vi "FRCts20_Backend_Test_Comment_GET.vi"(8 "error in (no error)":errorcluster, 11 "Note Index":u32) -> (0 "error out":errorcluster, 1 "Time (ms)":u32, 2 "Status":string, 3 "Note Out":T1, 5 "Success":bool)   [LabVIEW 2013, in "FRCts20_Backend_TestCode.lvlib"]
uses:
  FRCts20_Backend_TestCode.lvlib
  FRCts20_Backend_API/FRCts20_Backend_API_Note.ctl
  FRCts20_Backend_API/FRCts20_Backend_API_Command_Note.ctl
  FRCts20_Backend_API/FRCts20_Backend_API_Comment.vi
  FRCts20_Backend_API/FRCts20_Backend_API.lvlib
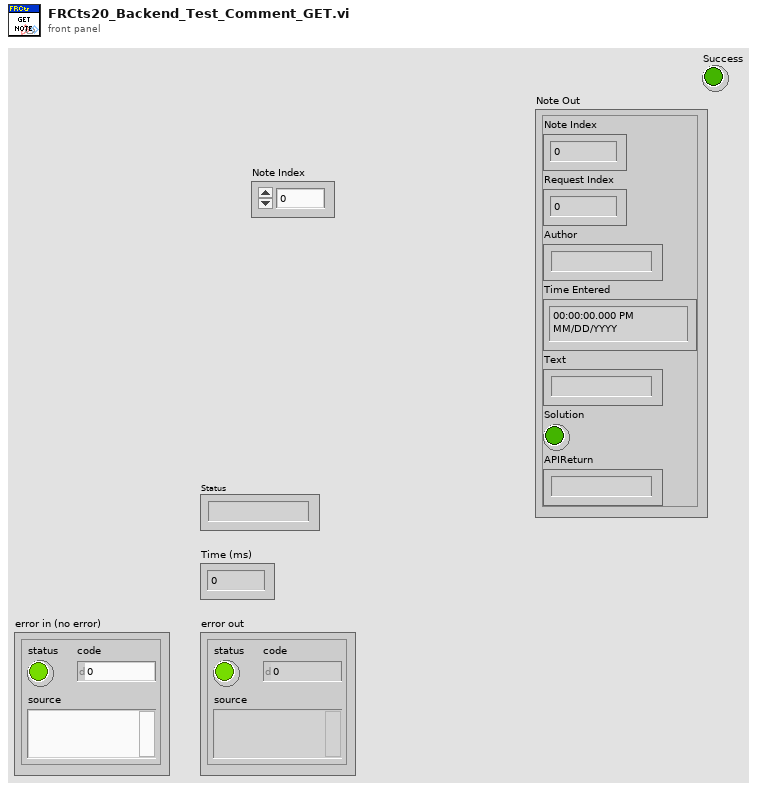
[diagram p1: front panel]
types:
  T1 = typedef "FRCts20_Backend_API.lvlib/FRCts20_Backend_API_Note.ctl" = cluster{"Note Index":u32, "Request Index":u32, "Author":string, "Time Entered":timestamp, "Text":string, "Solution":bool, "APIReturn":string}
  T2 = typedef "FRCts20_Backend_API.lvlib/FRCts20_Backend_API_Command_Note.ctl" = string
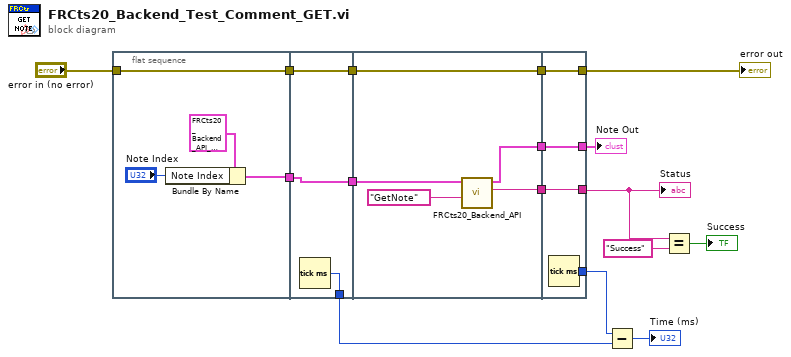
[diagram p0: block diagram]
diagram:
  n1 = flat-sequence {
    tunnel: [w20] -> w16
    tunnel: "error in (no error)" -> [w19]
    tunnel: [w19] -> w15
    tunnel: w16 -> [w21]
    tunnel: [w23] -> w8
    tunnel: [w22] -> w14
    tunnel: w15 -> [w22]
    tunnel: [w21] -> w2
    tunnel: [w28] -> w13
    tunnel: [w27] -> w12
    tunnel: [w26] -> w11
    tunnel: w14 -> [w26]
    tunnel: w2 -> [w24]
    tunnel: w13 -> [w32]
    tunnel: w12 -> [w31]
    tunnel: [w32] -> w5
    tunnel: [w31] -> w1
    tunnel: [w30] -> w7
    tunnel: [w29] -> w10
    tunnel: w11 -> [w29]
    frame #0 {
      n2 = Bundle By Name(cluster=T1 {"Note Index"=0, "Request Index"=0, "Author"="", "Time Entered"=timestamp(0 s since 1904-01-01), "Text"="", "Solution"=FALSE, "APIReturn"=""} ("Note In"), "Note Index"="Note Index") -> (w20:T1)
    }
    frame #1 {
      n3 = Tick Count (ms)() -> (millisecond timer value=w23:u32)
    }
    frame #2 {
      n4 = call-poly "FRCts20_Backend_API.vi"("Command"=T2 "GetNote", "Note In"=w24) -> ("Status"=w28:string, "Note Out"=w27:T1)  [unwired: 7 in, 1 out]
    }
    frame #3 {
      n5 = Tick Count (ms)() -> (millisecond timer value=w30:u32)
    }
  }
  n6 = Subtract(x=w7, y=w8) -> (x-y=→"Time (ms)":u32)
  n7 = Equal?(x=w5, y="Success") -> (x = y?=→"Success":bool)
  "error out" <- w10
  "Status" <- w5
  "Note Out" <- w1
